vi "Create Operation.vi"(0 "reference in":refnum<class "Factory.lvclass">, 5 "error in (no error)":errorcluster, 6 "Operation":enum16{"Add", "Mul"}(ring)) -> (14 "reference out":refnum<class "Factory.lvclass">, 16 "Operation":refnum<class "Operation.lvclass">, 19 "error out":errorcluster)   [LabVIEW 2013, in "Factory.lvclass"]
uses:
  Factory.lvclass
  Operation_class/Operation.lvclass
  Add_class/Add.lvclass
  Mul_class/Mul.lvclass
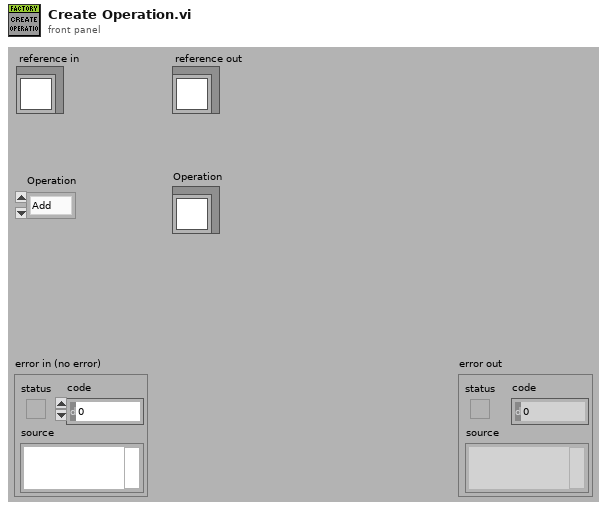
[diagram p1: front panel]
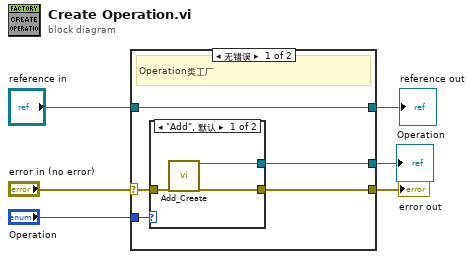
[diagram p0: block diagram]
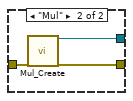
[diagram p2: hidden frame]
diagram:
  n1 = case shown="无错误" "error in (no error)" {
    selector: "error in (no error)" -> [w9 w19]
    tunnel: [w8 w19] -> w5
    tunnel: [w11 w18] -> w3
    tunnel: "reference in" -> [w11 w18]
    tunnel: "Operation" -> [w10 _]
    tunnel: [w7 _] -> w1
    frame No Error {
      # "Operation类工厂"
      n2 = case shown="\"Add\", 默认" w10 {
        tunnel: [w14 w17] -> w7
        tunnel: w9 -> [w13 w16]
        tunnel: [w12 w15] -> w8
        frame "Add", Default {
          n3 = call "Add_Create.vi"("error in (no error)"=w13) -> ("reference out"=w14:refnum<class "Add.lvclass">, "error out"=w12:errorcluster)  [unwired: 17 in]
        }
        frame "Mul" {
          n4 = call "Mul_Create.vi"("error in (no error)"=w16) -> ("reference out"=w17:refnum<class "Mul.lvclass">, "error out"=w15:errorcluster)  [unwired: 17 in]
        }
      }
    }
    frame Error {
    }
  }
  "error out" <- w5
  "reference out" <- w3
  "Operation" <- w1
